vi "Subtract.vi"(1 "x":sgl, 2 "y":sgl, 4 "Subtractor4":refnum<class "Subtractor4.lvclass">) -> (6 "x-y":sgl)   [LabVIEW 2017, in "Subtractor4.lvclass"]
uses:
  Subtractor4.lvclass
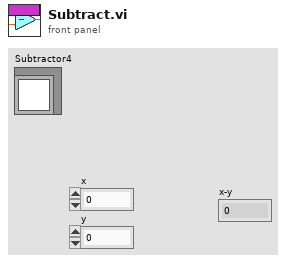
[diagram p1: front panel]
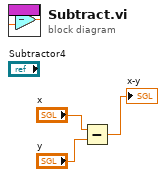
[diagram p0: block diagram]
diagram:
  n1 = Subtract(x="x", y="y") -> (x-y=→"x-y":sgl)
